vi "Main.vi"(0 "PID On":bool) -> (5 "Total (V)":dbl[](array[slide]) scale=-8.0..8.0, 6 "Force (N)":T2(graph)={"M1 ref force"=19.690402476780186, "M2 ref force"=19.690402476780186, "M1 mes force"=5.466389475814116, "M2 mes force"=1.4423805363163493})   [LabVIEW 2021]
uses:
  <vilib>/Platform/TimedLoop/XDataNode/timing_clust.ctl
  <vilib>/Platform/TimedLoop/XDataNode/nitl_modes.ctl
  <vilib>/Platform/TimedLoop/XDataNode/wakeup.ctl
  <vilib>/Analysis/baseanly.llb/Real Dot Product.vi
  <vilib>/DAQmx/write.llb/DAQmx Write (Digital 1D Bool 1Chan 1Samp).vi
  <vilib>/DAQmx/write.llb/DAQmx Write (Analog 1D DBL NChan 1Samp).vi
  <vilib>/DAQmx/create/channels.llb/DAQmx Create Channel (DO-Digital Output).vi
  <vilib>/DAQmx/create/channels.llb/DAQmx Create Channel (AO-Voltage-Basic).vi
  <vilib>/DAQmx/create/channels.llb/DAQmx Create Channel (AI-Voltage-Basic).vi
  <vilib>/addons/control/pid/pid.llb/PID (DBL).vi
  <vilib>/DAQmx/miscellaneous.llb/DAQmx Fill In Error Info.vi
  <vilib>/platform/TimedLoop/XDataNode/XDataNode.xnode
  <vilib>/addons/control/pid/NI_PID_pid.lvlib
  <vilib>/Platform/TimedLoop/XDataNode/XDNodeRunTimeDep.lvlib
  <vilib>/Analysis/NI_AALBase.lvlib
panel:
  in  "operation (0:open)":T1(ring)
  in  "stop 2":bool
  out "i":i32
  in  "Tab Control 2":enum32{"Start", "Trajectory", "RBF"}(tab)
  in  "Encoder":bool
  in  "Loadcell":bool
  in  "Set Tension":dbl=7.0
  in  "Motor Enable":bool[](array[boolean])=[FALSE, FALSE]
  in  "x":cluster{"Number":i32, "x_0":dbl, "x_f":dbl}={"Number"=20, "x_0"=0.0, "x_f"=500.0}
  in  "RBF":cluster{"STD":dbl, "Number":i32}={"STD"=150.0, "Number"=3}
  out "Weights":dbl[](array[numeric])=[3.49, 8.71, 7.36]
  out "Output":dbl(slide)=5.690310910676771 scale=0.0..10.0
  in  "Traj Start":i32(knob) scale=0.0..2.0
  in  "Tab Control":enum32{"Page 1", "Page 2"}(tab)
  out "XY Graph":cluster{dbl[], dbl[]}[](graph)=[{[0.0, 26.31578947368421, 52.63157894736842, 78.94736842105263, 105.26315789473684, 131.57894736842104, 157.89473684210526, 184.21052631578945, 210.52631578947367, 236.8421052631579, 263.1578947368421, 289.4736842105263, 315.7894736842105, 342.10526315789474, 368.4210526315789, 394.7368421052631, 421.05263157894734, 447.36842105263156, 473.6842105263158, 499.99999999999994], [3.49, 3.4367023266816097, 3.2816434014183695, 3.038602121132399, 2.728282054650678, 2.375405053956736, 2.0054833734466047, 1.6418498415053318, 1.303409208366113, 1.0033700058366293, 0.7489872481878055, 0.5421515616003525, 0.3805397094919775, 0.25900743528896036, 0.1709454164658713, 0.10940462192952286, 0.06789641734177898, 0.040859309931447936, 0.023843399552483855, 0.013492061286760112]}, {[0.0, 26.31578947368421, 52.63157894736842, 78.94736842105263, 105.26315789473684, 131.57894736842104, 157.89473684210526, 184.21052631578945, 210.52631578947367, 236.8421052631579, 263.1578947368421, 289.4736842105263, 315.7894736842105, 342.10526315789474, 368.4210526315789, 394.7368421052631, 421.05263157894734, 447.36842105263156, 473.6842105263158, 499.99999999999994], [2.1718577384502504, 2.86506550054527, 3.664972461281408, 4.546109122932967, 5.4681696051074065, 6.377890766498874, 7.213485399786169, 7.9112701950597755, 8.413568935864594, 8.676554069284796, 8.676554069284796, 8.413568935864594, 7.911270195059776, 7.213485399786169, 6.377890766498877, 5.468169605107408, 4.546109122932969, 3.6649724612814083, 2.86506550054527, 2.1718577384502518]}, {[0.0, 26.31578947368421, 52.63157894736842, 78.94736842105263, 105.26315789473684, 131.57894736842104, 157.89473684210526, 184.21052631578945, 210.52631578947367, 236.8421052631579, 263.1578947368421, 289.4736842105263, 315.7894736842105, 342.10526315789474, 368.4210526315789, 394.7368421052631, 421.05263157894734, 447.36842105263156, 473.6842105263158, 499.99999999999994], [0.028453172226519864, 0.050282928569135, 0.08616748455457215, 0.14318556780386613, 0.23072149495738908, 0.3605038009136996, 0.5462162532168332, 0.8025135420805027, 1.1433339522574764, 1.5795261165221341, 2.1159894678961577, 2.748736897872375, 3.462468433661673, 4.22932883340029, 5.009450199748302, 5.753626338747561, 6.408054903018468, 6.920600411014096, 7.247601468302764, 7.36]}, {[0.0, 26.31578947368421, 52.63157894736842, 78.94736842105263, 105.26315789473684, 131.57894736842104, 157.89473684210526, 184.21052631578945, 210.52631578947367, 236.8421052631579, 263.1578947368421, 289.4736842105263, 315.7894736842105, 342.10526315789474, 368.4210526315789, 394.7368421052631, 421.05263157894734, 447.36842105263156, 473.6842105263158, 499.99999999999994], [5.690310910676771, 6.352050755796014, 7.03278334725435, 7.727896811869232, 8.427173154715474, 9.11379962136931, 9.765185026449608, 10.35563357864561, 10.860312096488185, 11.259450191643559, 11.54153078536876, 11.704457395337322, 11.754278338213426, 11.701821668475418, 11.55828638271305, 11.331200565784492, 11.022060443293217, 10.626432182226953, 10.136510368400518, 9.545349799737012]}]
  out "Position (mm)":cluster{"Position":dbl, "ref_x (mm)":dbl}(graph)={"Position"=75.7275182286212, "ref_x (mm)"=0.0}
  out "dt":u32=4
  in  "RBF":bool
  out "Speed (RPM)":dbl[](array[knob]) scale=-200.0..200.0
  in  "Set Point":dbl(slide)=19.690402476780186 scale=0.0..40.0
  in  "stop":bool
  in  "Tab Control 3":enum32{"Page 1", "Page 3", "Page 4", "Page 2"}(tab)=enum."Page 2"
  in  "PID gains":T3 {"derivative time (Td, min)" format="%.3f"; "integral time (Ti, min)" format="%.3f"; "proportional gain (Kc)" format="%.3f"}
  in  "Pos Control":bool
  out "output":dbl(knob)=-0.0 scale=-40.0..40.0
  in  "Gains":T4(array[cluster])=[{"proportional gain (Kc)"=0.17, "integral time (Ti, min)"=0.0, "derivative time (Td, min)"=0.0}, {"proportional gain (Kc)"=0.17, "integral time (Ti, min)"=0.0, "derivative time (Td, min)"=0.0}] {"derivative time (Td, min)" format="%.3f"; "integral time (Ti, min)" format="%.3f"; "proportional gain (Kc)" format="%.3f"}
  out "PID (V)":dbl[](array[slide])=[2.4180822101642323, 1.0] scale=-8.0..8.0
  # "FORCE"
  # "TRAJECTORY"
  # "INITIALIZE"
  # "TUNE"
  # "MONITOR"
  # "DEVEL"
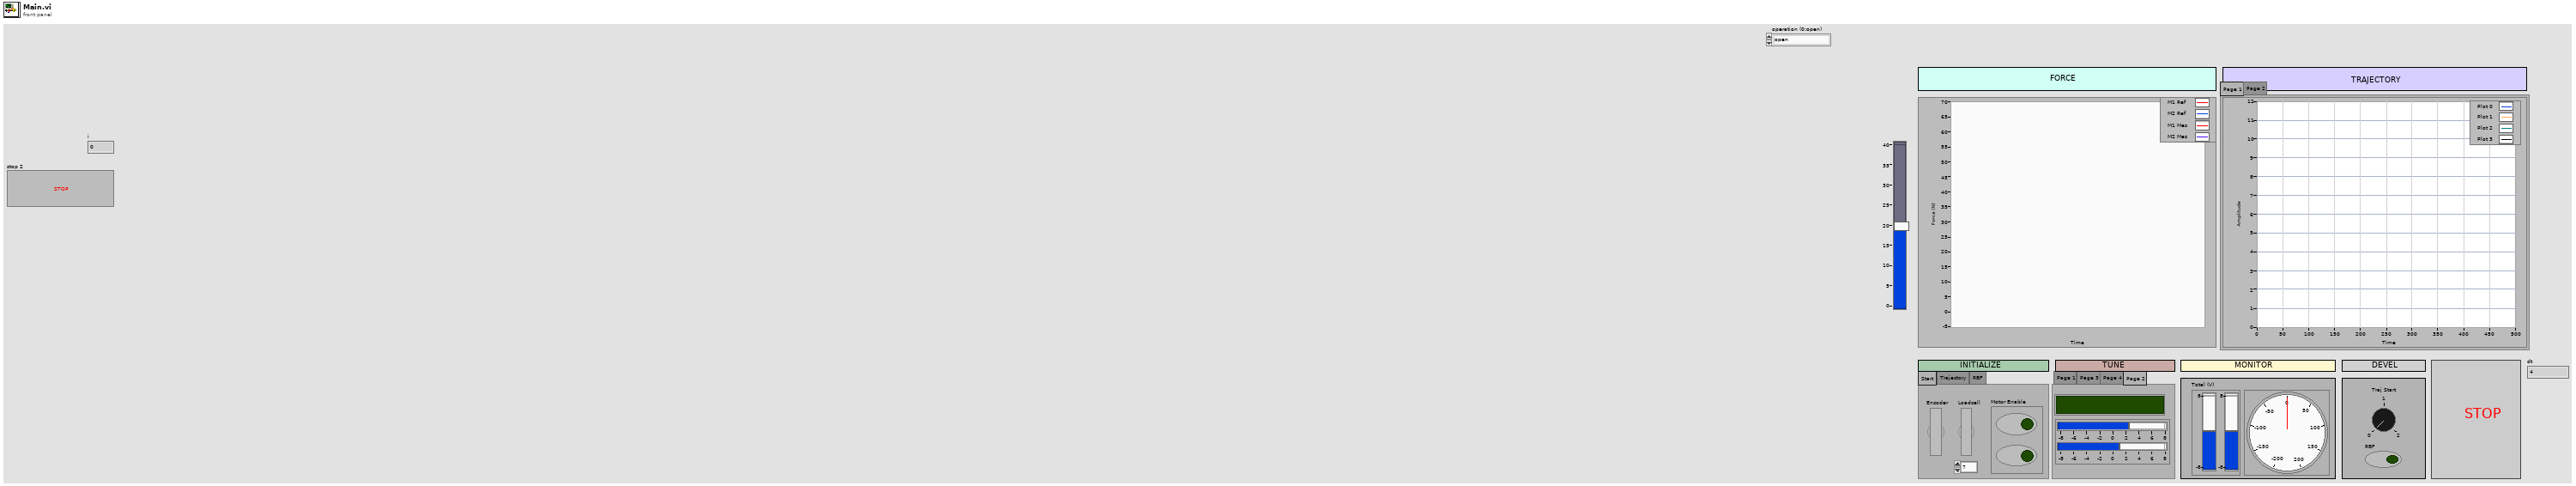
[diagram p1: front panel]
types:
  T1 = enum16{"open", "open or create", "create or replace", "create", "open (read-only)"}
  T2 = cluster{"M1 ref force":dbl, "M2 ref force":dbl, "M1 mes force":dbl, "M2 mes force":dbl}
  T3 = cluster{"proportional gain (Kc)":dbl, "integral time (Ti, min)":dbl, "derivative time (Td, min)":dbl}
  T4 = cluster{"proportional gain (Kc)":dbl, "integral time (Ti, min)":dbl, "derivative time (Td, min)":dbl}[]
  T5 = typedef "XDNodeRunTimeDep.lvlib/timing_clust.ctl" = cluster{"Expected End [f-1]":u64, "Actual End [f-1]":u64, "Finished Late? [f-1]":bool, "Expected End [i-1]":u64, "Actual End [i-1]":u64, "Finished Late? [i-1]":bool, "Expected Start [i]":u64, "Actual Start [i]":u64, "Expected Start [f]":u64, "Actual Start [f]":u64, "Source Name":string, "Structure Name":string, "Period":i64, "Deadline":i64, "Offset":i64, "Start":i64, "Priority":i32, "Timeout":i32, "Mode":T6, "Wakeup Reason":T7, "Error":errorcluster, "Source Type":string, "Secondary Source Type":string, "Global End Time":u64, "Global Start Time":u64, "Frame Duration":u64, "Iteration Duration":u64, "Assigned CPU":i32, "I/O Scan Engine Mode":u32}
  T6 = typedef "XDNodeRunTimeDep.lvlib/nitl_modes.ctl" = enum32{"No Change", "Process missed periods, maintain original phase", "Discard missed periods, maintain original phase", "Process missed periods, ignore original phase", "Discard missed periods, ignore original phase"}
  T7 = typedef "XDNodeRunTimeDep.lvlib/wakeup.ctl" = enum32{"Normal", "Aborted", "Asynchronous wakeup", "Timing source error", "Timed loop error", "Timeout"}
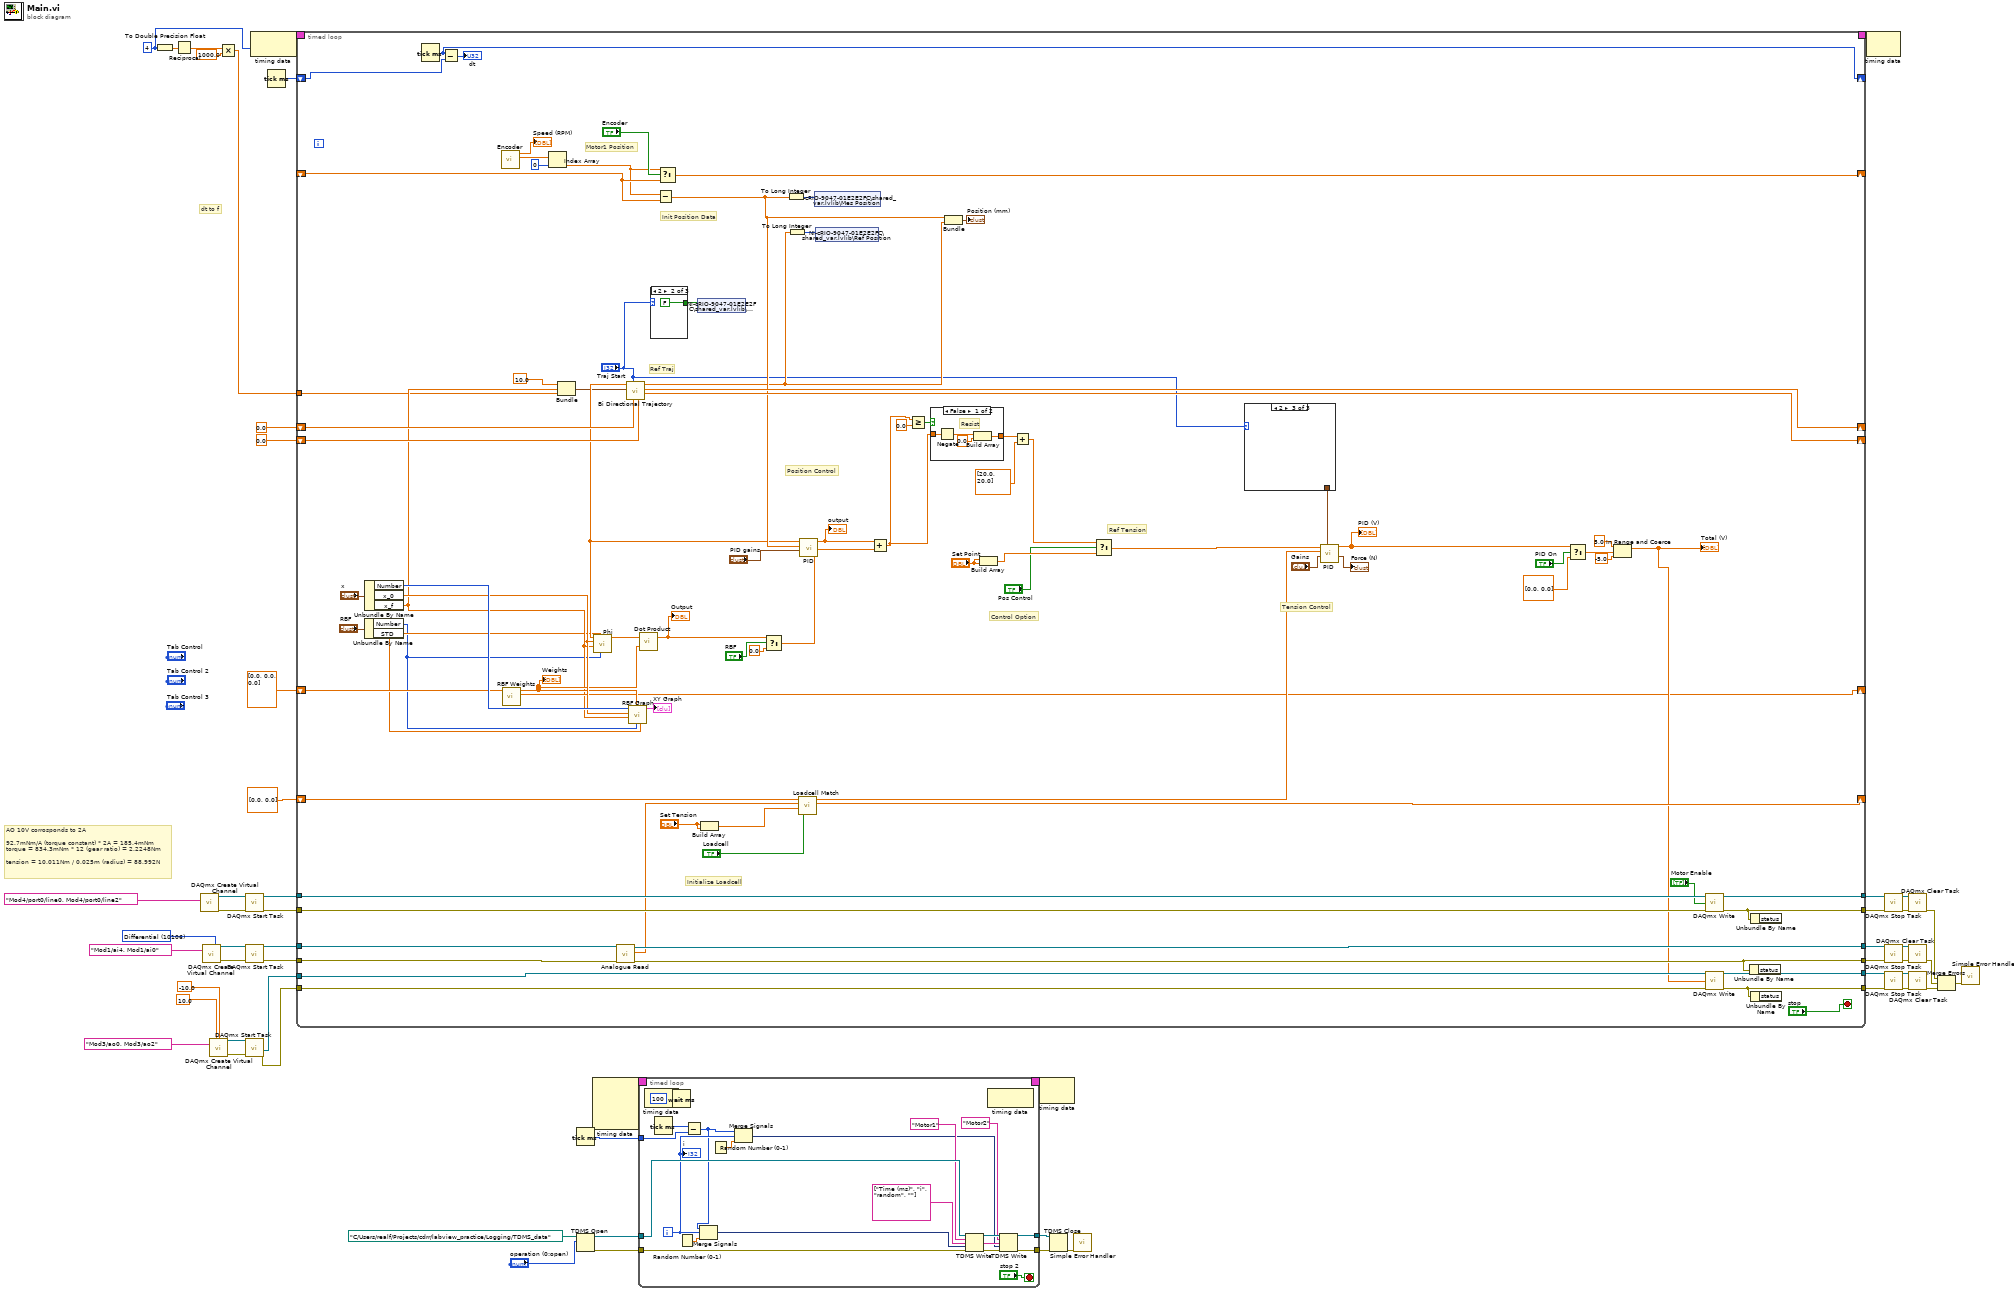
[diagram p0: block diagram]
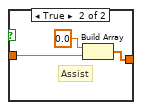
[diagram p2: hidden frame]
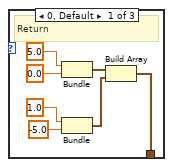
[diagram p3: hidden frame]
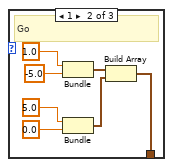
[diagram p4: hidden frame]
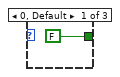
[diagram p5: hidden frame]
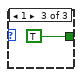
[diagram p6: hidden frame]
diagram:
  w15 = i64 4 ("Period")
  w23 = 10106 items=["Default"=-1, "RSE"=10083, "NRSE"=10078, "Differential"=10106, "Pseudodifferential"=12529] ("input terminal configuration")
  # "dt to f"
  # "AO 10V corrosponds to 2A\n\n92.7mNm/A (torque constant) * 2A = 185.4mNm\ntorque = 834.3mNm * 12 (gear ratio) = 2.2248Nm\n\ntension = 10.011Nm / 0.025m (radius) = 88.992N"
  n1 = To Double Precision Float(number=w15) -> (double precision float=w14:dbl)
  n2 = Reciprocal(x=w14) -> (1/x=w13:dbl)
  n3 = call-poly <vilib>:"DAQmx Create Virtual Channel.vi"("lines"=tag "Mod4/port0/line0, Mod4/port0/line2") -> ("task out"=w50:refnum<k21>, "error out"=w49:errorcluster)  [unwired: 13 in]
  n4 = call-poly <vilib>:"DAQmx Create Virtual Channel.vi"("input terminal configuration"=w23, "physical channels"=tag "Mod1/ai4, Mod1/ai0") -> ("task out"=w40:refnum<k21>, "error out"=w41:errorcluster)  [unwired: 12 in]
  n5 = call-poly <vilib>:"DAQmx Create Virtual Channel.vi"("maximum value"=10.0 ("AO max"), "minimum value"=-10.0 ("AO min"), "physical channels"=tag "Mod3/ao0, Mod3/ao2" ("Physical Channel(s)")) -> ("task out"=w34:refnum<k21>, "error out"=w33:errorcluster)  [unwired: 11 in]
  n6 = Multiply(x=w13, y=1000.0) -> (x*y=w11:dbl)
  n7 = call <vilib>:"DAQmx Start Task.vi"("task/channels in"=w50, "error in"=w49) -> ("task out"=w47:refnum<k21>, "error out"=w46:errorcluster)  [unwired: 12 in]
  n8 = call <vilib>:"DAQmx Start Task.vi"("task/channels in"=w40, "error in"=w41) -> ("task out"=w38:refnum<k21>, "error out"=w37:errorcluster)  [unwired: 12 in]
  n9 = call <vilib>:"DAQmx Start Task.vi"("task/channels in"=w34, "error in"=w33) -> ("task out"=w52:refnum<k21>, "error out"=w51:errorcluster)  [unwired: 12 in]
  n10 = node-c288(w15) -> (w18:T5)
  n11 = Tick Count (ms)() -> (millisecond timer value=w19:u32)
  n12 = timed-loop {
    tunnel: [w139] -> w56
    tunnel: [w138] -> w55
    tunnel: [w125] -> w54
    tunnel: [w130] -> w53
    tunnel: w38 -> [w136]
    tunnel: w37 -> [w135]
    tunnel: w52 -> [w124]
    tunnel: w51 -> [w137]
    tunnel: w47 -> [w134]
    tunnel: w46 -> [w133]
    tunnel: [w132] -> w43
    tunnel: [w131] -> w42
    shift-right: [w128] -> _
    shift-left: 0.0 ("total time") -> [w129]
    shift-right: [w127] -> _
    shift-left: _ -> [w126]
    shift-right: [w122] -> _
    shift-left: dbl[] [0.0, 0.0] ("measured force") -> [w123]
    shift-right: [w120] -> _
    shift-left: 0.0 ("total time") -> [w121]
    timing: w18 -> [_]
    timing-out: [_] -> w17
    shift-right: [w91] -> _
    shift-left: w19 -> [w93]
    shift-right: [w71] -> _
    shift-left: dbl[] [0.0, 0.0, 0.0] ("Array of Double") -> [w72]
    tunnel: w11 -> [w61]
    stop <- "stop" stop-if-true
    # "Initialize Loadcell"
    # "Tension Control"
    # "Ref Tension"
    # "Position Control"
    # "Ref Traj"
    # "Control Option"
    # "Init Position Data"
    # "Motor1 Position"
    n13 = Unbundle By Name("RBF") -> ("Number"=w57:i32, "STD"=w58:dbl)
    n14 = Unbundle By Name("x") -> ("Number"=w81:i32, "x_0"=w78:dbl, "x_f"=w62:dbl)
    n15 = Tick Count (ms)() -> (millisecond timer value=w91:u32)
    n16 = Subtract(x=w91, y=w93) -> (x-y=→"dt":u32)
    n17 = call "Encoder.vi"() -> ("Mes Pos (mm)"=w85:dbl[], "RPM"=→"Speed (RPM)":dbl[])  [unwired: 10 in]
    n18 = call "RBF Weights.vi"("Array of Double in"=w72) -> ("Array of Double out"=w71:dbl[], "Array of Double 3"=w73:dbl[])  [unwired: 9 in]
    "Weights" <- w73
    n19 = Index Array(array=w85, index=0) -> (element=w102:dbl)
    n20 = Bundle("y"=10.0, "x_f"=w62, w61) -> (w60:cluster{"y":dbl, "x_f":dbl, dbl})  [unwired: 1 in]
    n21 = call "Analogue Read.vi"("error in"=w135, "task/channels in"=w136) -> ("error out"=w130:errorcluster, "measured force"=w96:dbl[], "task out"=w125:refnum<k21>)  [unwired: 6 in, 1 out]
    n22 = call "Bi Directional Trajectory.vi"("Return Time"=w121, "Go Time"=w129, "Traj Start"="Traj Start", "Trajectory Settings"=w60) -> ("Return Next Time"=w120:dbl, "Go Next Time"=w128:dbl, "Output (mm)"=w77:dbl)  [unwired: 5 in]
    n23 = call "Phi.vi"("Number"=w57, "STD"=w58, "x_f"=w62, "x_0"=w78, "Output (mm)"=w77) -> ("Array"=w76:dbl[])  [unwired: 6 in]
    n24 = call "RBF Graph.vi"("STD"=w58, "Number"=w57, "Array of Double 3"=w73, "x_f"=w62, "x_0"=w78, "Number 2"=w81) -> ("Array"=→"XY Graph":cluster{dbl[], dbl[]}[])  [unwired: 5 in]
    n25 = call-poly <vilib>:"Dot Product.vi"("Y Vector"=w73, "X Vector"=w76) -> ("X * Y"=w70:dbl)  [unwired: 1 out]
    "Output" <- w70
    n26 = case shown="2" "Traj Start" {
      tunnel: [FALSE FALSE TRUE] -> w74
      frame 0, Default {
      }
      frame 2 {
      }
      frame 1 {
      }
    }
    n27 = Subtract(x=w102, y=w126) -> (x-y=w104:dbl)
    n28 = Select(t=w102, s="Encoder", f=w126) -> (s? t:f=w127:dbl)
    n29 = shared-variable "NI-cRIO-9047-01E2E2FC\\shared_var.lvlib\\Trigger"(w74) -> ()  [unwired: 1 in, 1 out]
    n30 = Build Array("Set Tension", "Set Tension") -> (w94:dbl[])
    n31 = Select(t=w70, s="RBF", f=0.0) -> (s? t:f=w99:dbl)
    n32 = To Long Integer(number=w104) -> (32bit integer=w87:i32)
    n33 = To Long Integer(number=w77) -> (32bit integer=w88:i32)
    n34 = call "Loadcell Match.vi"("Initialize"="Loadcell", "Set Tension"=w94, "Mes Tension"=w96, "Next Tension Error"=w123) -> ("Tension Error"=w122:dbl[], "Filtered Tension"=w106:dbl[])  [unwired: 6 in]
    n35 = call-poly <vilib>:"PID.vi"("PID gains"="PID gains", "process variable"=w104, "setpoint"=w77) -> ("output"=w63:dbl)  [unwired: 7 in, 1 out]
    "output" <- w63
    n36 = shared-variable "NI-cRIO-9047-01E2E2FC\\shared_var.lvlib\\Mes Position"(w87) -> ()  [unwired: 1 in, 1 out]
    n37 = shared-variable "NI-cRIO-9047-01E2E2FC\\shared_var.lvlib\\Ref Position"(w88) -> ()  [unwired: 1 in, 1 out]
    n38 = Add(x=w63, y=w99) -> (x+y=w65:dbl)
    n39 = Greater Or Equal?(x=w65, y=0.0) -> (x >= y?=w69:bool)
    n40 = case shown="False" w69 {
      tunnel: w65 -> [w142 w145]
      tunnel: [w143 w146] -> w66
      frame False {
        # "Resist"
        n41 = Negate(x=w142) -> (-x=w140:dbl)
        n42 = Build Array(w140, 0.0 ("element")) -> (w143:dbl[])
      }
      frame True {
        # "Assist"
        n43 = Build Array(0.0 ("element"), w145) -> (w146:dbl[])
      }
    }
    n44 = Bundle(w104, "Output (mm)"=w77) -> (→"Position (mm)":cluster{dbl, "Output (mm)":dbl})  [unwired: 1 in]
    n45 = Build Array("Set Point", "Set Point") -> (w112:dbl[])
    n46 = Add(x=w66, y=dbl[] [20.0, 20.0] ("x")) -> (x+y=w64:dbl[])
    n47 = Select(t=w64, s="Pos Control", f=w112) -> (s? t:f=w100:dbl[])
    n48 = case shown="2" "Traj Start" {
      tunnel: [w147 w154 _] -> w107
      frame 0, Default {
        # "Return"
        n49 = Bundle(5.0, 0.0) -> (w153:cluster{dbl, dbl})  [unwired: 1 in]
        n50 = Bundle(1.0, -5.0) -> (w152:cluster{dbl, dbl})  [unwired: 1 in]
        n51 = Build Array(w153, w152) -> (w147:cluster{dbl, dbl}[])
      }
      frame 1 {
        # "Go"
        n52 = Bundle(1.0, -5.0) -> (w155:cluster{dbl, dbl})  [unwired: 1 in]
        n53 = Bundle(5.0, 0.0) -> (w156:cluster{dbl, dbl})  [unwired: 1 in]
        n54 = Build Array(w155, w156) -> (w154:cluster{dbl, dbl}[])
      }
      frame 2 {
      }
    }
    n55 = call <vilib>:"PID.vi"("output range"=w107, "PID gains"="Gains", "mes force"=w106, "ref force"=w100) -> ("output cluster"=→"Force (N)":T2, "PID output"=w116:dbl[])  [unwired: 6 in]
    "PID (V)" <- w116
    n56 = Select(t=w116, s="PID On", f=dbl[] [0.0, 0.0]) -> (s? t:f=w114:dbl[])
    n57 = In Range and Coerce(upper limit=5.0, x=w114, lower limit=-5.0) -> (coerced(x)=w89:dbl[])  [unwired: 1 out]
    "Total (V)" <- w89
    n58 = call-poly <vilib>:"DAQmx Write.vi"("task/channels in"=w134, "data"="Motor Enable", "error in"=w133) -> ("task out"=w132:refnum<k21>, "error out"=w131:errorcluster)  [unwired: 10 in, 1 out]
    n59 = call-poly <vilib>:"DAQmx Write.vi"("task/channels in"=w124, "data"=w89, "error in"=w137) -> ("task out"=w139:refnum<k21>, "error out"=w138:errorcluster)  [unwired: 10 in, 1 out]
    n60 = Unbundle By Name(w130) -> ()  [unwired: 1 out]
    n61 = Unbundle By Name(w131) -> ()  [unwired: 1 out]
    n62 = Unbundle By Name(w138) -> ()  [unwired: 1 out]
  }
  n63 = Tick Count (ms)() -> (millisecond timer value=w3:u32)
  n64 = TDMS Open(10:"operation (0:open)", 11:path "C:/Users/realf/Projects/cdrr/labview_practice/Logging/TDMS_data" ("file path")) -> (0:w6:errorcluster, 3:w10:refnum<k34>)  [unwired: 5 in]
  n65 = node-c288() -> (w2:T5)  [unwired: 4 in]
  n66 = timed-loop {
    tunnel: w10 -> [w183]
    tunnel: [w177] -> w9
    tunnel: [w179] -> w7
    tunnel: w6 -> [w182]
    tunnel: w3 -> [w167]
    timing: w2 -> [_]
    timing-out: [_] -> w1
    i -> [w168]
    stop <- "stop 2" stop-if-true
    n67 = node-c288() -> ()  [unwired: 1 in, 1 out]
    n68 = Tick Count (ms)() -> (millisecond timer value=w170:u32)
    n69 = Wait (ms)(milliseconds to wait=u32 100) -> ()  [unwired: 1 out]
    n70 = Random Number (0-1)() -> (number: 0 to 1=w169:dbl)
    n71 = Subtract(x=w170, y=w167) -> (x-y=w166:u32)
    n72 = Merge Signals(w166, w168, w169) -> (w173:dynamicdata)
    n73 = Random Number (0-1)() -> (number: 0 to 1=w172:dbl)
    n74 = Merge Signals(w166, w168, w172) -> (w171:dynamicdata)
    n75 = TDMS Write(0:w183, 5:"Motor1" ("group name in (Untitled)"), 7:string[] ["Time (ms)", "i", "random", ""] ("channel name(s) in (Untitled)"), 9:w173, 11:w182) -> (4:w178:refnum<k34>, 8:w174:string[], 15:w180:errorcluster)  [unwired: 1 in, 1 out]
    n76 = node-c288() -> ()  [unwired: 1 in, 1 out]
    n77 = TDMS Write(0:w178, 5:"Motor2" ("group name in (Untitled)"), 7:w174, 9:w171, 11:w180) -> (4:w177:refnum<k34>, 15:w179:errorcluster)  [unwired: 1 in, 2 out]
    "i" <- w168
  }
  n78 = node-c288(w1) -> ()  [unwired: 1 out]
  n79 = TDMS Close(8:w7, 11:w9) -> (0:w8:errorcluster)  [unwired: 1 out]
  n80 = call <vilib>:"Simple Error Handler.vi"("error in (no error)"=w8) -> ()  [unwired: 4 in, 5 out]
  n81 = node-c288(w17) -> ()  [unwired: 1 out]
  n82 = call <vilib>:"DAQmx Stop Task.vi"("task/channels in"=w43, "error in"=w42) -> ("task out"=w45:refnum<k21>, "error out"=w44:errorcluster)  [unwired: 12 in]
  n83 = call <vilib>:"DAQmx Stop Task.vi"("task/channels in"=w54, "error in"=w53) -> ("task out"=w29:refnum<k21>, "error out"=w28:errorcluster)  [unwired: 12 in]
  n84 = call <vilib>:"DAQmx Stop Task.vi"("task/channels in"=w56, "error in"=w55) -> ("task out"=w31:refnum<k21>, "error out"=w30:errorcluster)  [unwired: 12 in]
  n85 = call <vilib>:"DAQmx Clear Task.vi"("task in"=w45, "error in"=w44) -> ("error out"=w24:errorcluster)  [unwired: 13 in]
  n86 = call <vilib>:"DAQmx Clear Task.vi"("task in"=w29, "error in"=w28) -> ("error out"=w25:errorcluster)  [unwired: 13 in]
  n87 = call <vilib>:"DAQmx Clear Task.vi"("task in"=w31, "error in"=w30) -> ("error out"=w26:errorcluster)  [unwired: 13 in]
  n88 = Merge Errors(w24, w25, w26) -> (w27:errorcluster)
  n89 = call <vilib>:"Simple Error Handler.vi"("error in (no error)"=w27) -> ()  [unwired: 4 in, 5 out]
